vi "labcontrol_gui.vi"() -> ()   [LabVIEW 2014]
uses:
  labcontrol.ctl
panel:
  in  "IP address":string="192.168.4.129"
  in  "Enum":T1(ring)
  out "command_debug":string
  out "error out":errorcluster
  out "data out":string
  in  "Channel Sequences":T3(array[cluster])=[{"Array"=[[0.0, 0.0], [0.0, 0.0], [0.0, 0.0], [4.0, 6.8789]], "enable"=TRUE, "initial [V / logic]"=3.0, "String"="CH 1"}, {"Array"=[[0.0, 0.0], [0.0, 0.0], [7.0, 0.0]], "enable"=TRUE, "initial [V / logic]"=99.0, "String"="CH 2"}, {"Array"=[], "enable"=FALSE, "initial [V / logic]"=0.0, "String"="LED 0"}, {"Array"=[], "enable"=FALSE, "initial [V / logic]"=0.0, "String"="LED 1"}, {"Array"=[], "enable"=FALSE, "initial [V / logic]"=0.0, "String"="LED 2"}, {"Array"=[], "enable"=FALSE, "initial [V / logic]"=0.0, "String"="LED 3"}, {"Array"=[], "enable"=FALSE, "initial [V / logic]"=0.0, "String"="LED 4"}, {"Array"=[], "enable"=FALSE, "initial [V / logic]"=0.0, "String"="LED 5"}, {"Array"=[], "enable"=FALSE, "initial [V / logic]"=0.0, "String"="LED 6"}, {"Array"=[], "enable"=FALSE, "initial [V / logic]"=0.0, "String"="LED 7"}, {"Array"=[], "enable"=FALSE, "initial [V / logic]"=0.0, "String"="EXP_P 0 (Trigger)"}, {"Array"=[], "enable"=FALSE, "initial [V / logic]"=0.0, "String"="EXP_P 1"}, {"Array"=[], "enable"=FALSE, "initial [V / logic]"=0.0, "String"="EXP_P 2"}, {"Array"=[], "enable"=FALSE, "initial [V / logic]"=0.0, "String"="EXP_P 3"}, {"Array"=[], "enable"=FALSE, "initial [V / logic]"=0.0, "String"="EXP_P 4"}, {"Array"=[], "enable"=FALSE, "initial [V / logic]"=0.0, "String"="EXP_P 5"}, {"Array"=[], "enable"=FALSE, "initial [V / logic]"=0.0, "String"="EXP_P 6"}, {"Array"=[], "enable"=FALSE, "initial [V / logic]"=0.0, "String"="EXP_P 7"}, {"Array"=[], "enable"=FALSE, "initial [V / logic]"=0.0, "String"="EXP_N 0"}, {"Array"=[], "enable"=FALSE, "initial [V / logic]"=0.0, "String"="EXP_N 1"}, {"Array"=[], "enable"=FALSE, "initial [V / logic]"=0.0, "String"="EXP_N 2"}, {"Array"=[], "enable"=FALSE, "initial [V / logic]"=0.0, "String"="EXP_N 3"}, {"Array"=[], "enable"=FALSE, "initial [V / logic]"=0.0, "String"="EXP_N 4"}, {"Array"=[], "enable"=FALSE, "initial [V / logic]"=0.0, "String"="EXP_N 5"}, {"Array"=[], "enable"=FALSE, "initial [V / logic]"=0.0, "String"="EXP_N 6"}, {"Array"=[], "enable"=FALSE, "initial [V / logic]"=0.0, "String"="EXP_N 7"}]
  # "Voltage [V] / \nlevel [logic]"
  # "Time [s]"
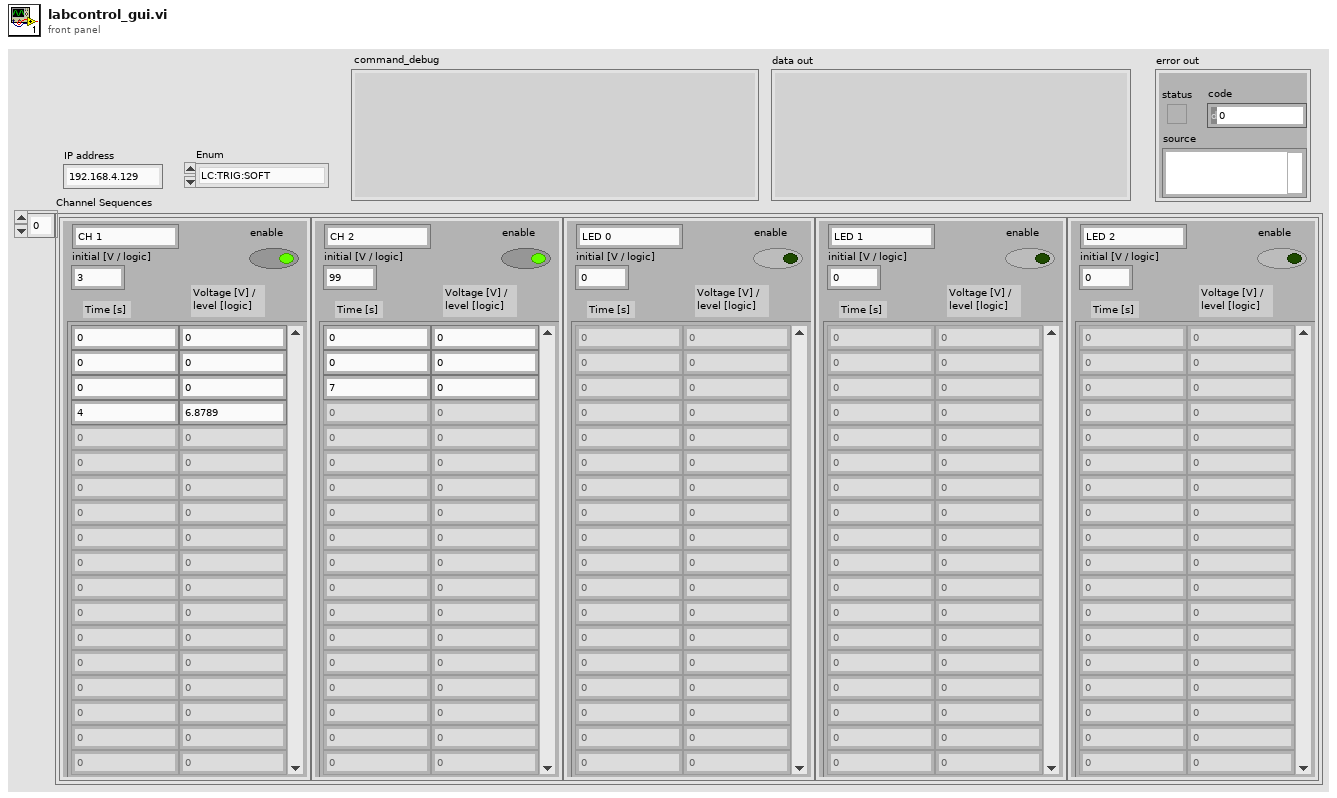
[diagram p1: front panel]
types:
  T1 = enum16{"LC:TRIG:SOFT", "LC:TRIG:AWAIT", "LC:DATA"}
  T2 = typedef "labcontrol.ctl" = dbl
  T3 = cluster{"Array":T2[][], "enable":bool, "initial [V / logic]":dbl, "String":string}[]
  T4 = cluster{"Array":T2[][], "initial [V / logic]":dbl, "enable":bool}
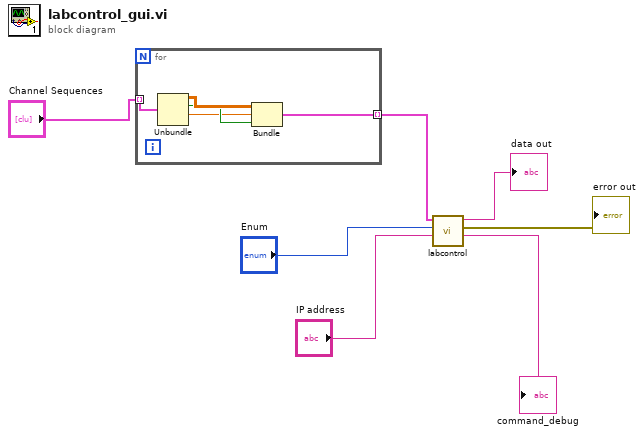
[diagram p0: block diagram]
diagram:
  n1 = for {
    tunnel: "Channel Sequences" -> [w12] mode=indexing
    tunnel: [w10] -> w6 mode=indexing
    n2 = Unbundle(w12) -> ("Array"=w11:T2[][], "enable"=w9:bool, "initial [V / logic]"=w8:dbl)  [unwired: 1 out]
    n3 = Bundle("Array"=w11, "initial [V / logic]"=w8, "enable"=w9) -> (w10:T4)  [unwired: 1 in]
  }
  n4 = call "labcontrol.vi"("IP address"="IP address", "Enum"="Enum", "data"=w6) -> ("command_debug"=→"command_debug":string, "error out"=→"error out":errorcluster, "data out"=→"data out":string)  [unwired: 6 in]
